vi "Is Point in Rect.vi"(10 "point":cluster{"x":i16, "y":i16}, 11 "rect":T1) -> (3 "Point in Rect?":bool)   [LabVIEW 2012]
doc: "Determines if a point is located inside a given rectangle"
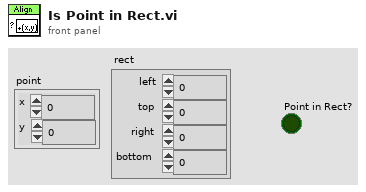
[diagram p1: front panel]
types:
  T1 = cluster{"left":i16, "top":i16, "right":i16, "bottom":i16}
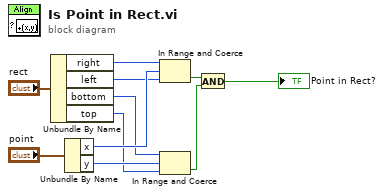
[diagram p0: block diagram]
diagram:
  n1 = Unbundle By Name("rect") -> ("right"=w3:i16, "left"=w7:i16, "bottom"=w1:i16, "top"=w2:i16)
  n2 = Unbundle By Name("point") -> ("x"=w11:i16, "y"=w10:i16)
  n3 = In Range and Coerce(upper limit=w3, x=w11, lower limit=w7) -> (In Range?=w9:bool)  [unwired: 1 out]
  n4 = In Range and Coerce(upper limit=w1, x=w10, lower limit=w2) -> (In Range?=w6:bool)  [unwired: 1 out]
  n5 = And(x=w9, y=w6) -> (x .and. y?=→"Point in Rect?":bool)
